vi "AlazarExtractNPTFootersExU16.vi"(0 "Buffer":u16[](array[numeric]), 5 "Options":T2={"Board Type"=29, "Domain"=4096, "Channel Count"=65536, "Data Layout"=3145728} {"Board Type" items=["ATS_NONE", "ATS850", "ATS310", "ATS330", "ATS855", "ATS315", "ATS335", "ATS460", "ATS860", "ATS660", "ATS665", "ATS9462", "ATS9434", "ATS9870", "ATS9350", "ATS9325", "ATS9440", "ATS9410", "ATS9351", "ATS9310", "ATS9461", "ATS9850", "ATS9625", "ATG6500", "ATS9626", "ATS9360", "AXI9870", "ATS9370", "ATU7825", "ATS9373", "ATS9416", "ATS9637", "ATS9120", "ATS9371", "ATS9130", "ATS9352", "ATS9453", "ATS9146", "ATS9000", "ATST371", "ATS9437", "ATS9618", "ATS9358"]; "Domain" items=["Time Domain"=4096, "Fourier Domain"=8192]; "Channel Count" items=["1 channel"=65536, "2 channels"=131072, "4 channels"=196608, "8 channels"=262144, "16 channels"=327680]; "Data Layout" items=["FFT"=0, "Buffer Interleaved"=1048576, "Record Interleaved"=2097152, "Sample Interleaved"=3145728]}, 7 "Record Size (bytes)":u32, 9 "Footers Count":u32, 11 "error in (no error)":errorcluster) -> (4 "footersArray":T1(array[cluster]), 10 "Return Code":u32, 15 "error out":errorcluster)   [LabVIEW 2009]
doc: "Configure a board to make an asynchronous AutoDMA acquisition."
uses:
  ATSApi.dll
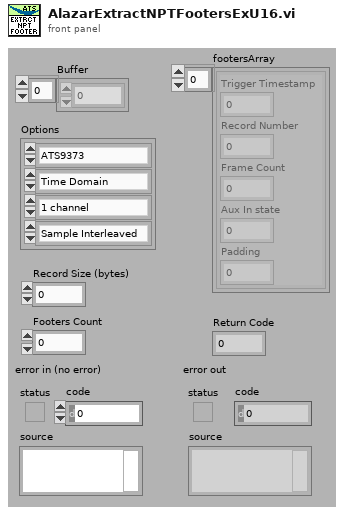
[diagram p1: front panel]
types:
  T1 = cluster{"Trigger Timestamp":u64, "Record Number":u32, "Frame Count":u32, "Aux In state":i32, "Padding":u32}[]
  T2 = cluster{"Board Type":u32, "Domain":u32, "Channel Count":u32, "Data Layout":u32}
  T3 = cluster{"Trigger Timestamp":u64, "Record Number":u32, "Frame Count":u32, "Aux In state":i32, "Padding":u32}
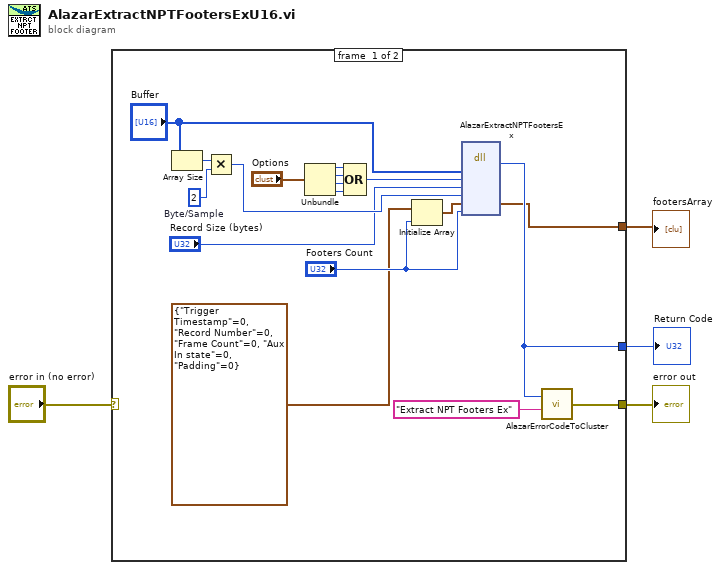
[diagram p0: block diagram]
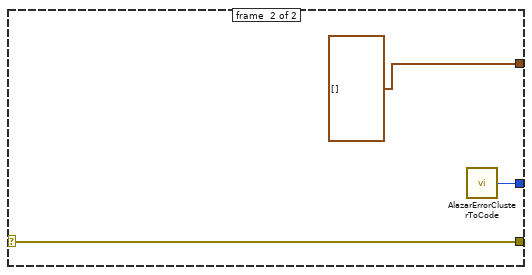
[diagram p2: hidden frame]
diagram:
  n1 = case shown="No Error" "error in (no error)" {
    selector: "error in (no error)" -> [_ w24]
    tunnel: [w20 w24] -> w4
    tunnel: [w22 w25] -> w3
    tunnel: [w5 T1 [] ("footersArray")] -> w1
    frame #0 {
      w12 = u32 2  # Byte/Sample
      n2 = Array Size(array="Buffer") -> (size(s)=w19:i32)
      n3 = Multiply(x=w19, y=w12) -> (x*y=w10:u32)
      n4 = Unbundle("Options") -> ("Board Type"=w18:u32, "Domain"=w17:u32, "Channel Count"=w16:u32, "Data Layout"=w15:u32)
      n5 = Compound Arithmetic op=OR(w18, w17, w16, w15) -> (w13:u32)
      n6 = Initialize Array(T3 {"Trigger Timestamp"=0, "Record Number"=0, "Frame Count"=0, "Aux In state"=0, "Padding"=0}, "Footers Count") -> (w9:T1)
      n7 = dll-call lib="ATSApi.dll" fn="AlazarExtractNPTFootersEx"("buffer"="Buffer", "options"=w13, "recordSize_bytes"="Record Size (bytes)", "bufferSize_bytes"=w10, "footersArray"=w9, "numFootersToExtract"="Footers Count") -> ("return type"=w22:u32, "footersArray"=w5:T1)  [unwired: 8 in, 2 out]
      n8 = call "AlazarErrorCodeToCluster.vi"("Message"="Extract NPT Footers Ex", "Error Code"=w22) -> ("error out"=w20:errorcluster)
    }
    frame #1 {
      n9 = call "AlazarErrorClusterToCode.vi"() -> ("Error Code"=w25:u32)  [unwired: 1 in]
    }
  }
  "error out" <- w4
  "Return Code" <- w3
  "footersArray" <- w1
